vi "Open Me.vi"   [LabVIEW 2019]
uses:
  <userlib>/LevyLab/Instrument Framework/Instrument Types/Cryostat/Instrument.Cryostat.lvclass
  <userlib>/LevyLab/Lockin-Multichannel/Instrument.DAQ/Typedefs/Sweep.Configuration--Cluster.ctl
  <userlib>/LevyLab/Lockin-Multichannel/Instrument.DAQ/Typedefs/Sweep.Channel--Cluster--Array.ctl
  <userlib>/LevyLab/Lockin-Multichannel/Instrument.DAQ/Typedefs/Sweep.Channel--Cluster.ctl
  <userlib>/LevyLab/Lockin-Multichannel/Instrument.DAQ/Typedefs/Sweep.Pattern--Enum.ctl
  SweepControl/Typedefs/ScanControl.ctl
  SweepControl/Typedefs/Cluster - ScanControl.ctl
  SweepControl/Typedefs/Enum - Priority.ctl
  SweepControl/Typedefs/Enum - Action.ctl
  SweepControl/Typedefs/ScanParamters.ctl
  SweepControl/Typedefs/Cluster - ScanParamters.ctl
  SweepControl/Typedefs/PostAction.ctl
  SweepControl/Typedefs/Enum - PostAction.ctl
  Control Experiment/Control Experiment.lvclass/Control Experiment.ctl
  Transport/Transport.lvclass/Transport.ctl
  SweepControl/SweepControl.lvclass/SweepControl.ctl
  1ef964a1-2c2c-4dd9-a479-5e3cab6bfeb3.vi
  Control Experiment/subVIs/String Label.vi
  Transport/Transport.lvclass
  Control Experiment/Control Experiment.lvclass
  SweepControl/SweepControl.lvclass
  <userlib>/LevyLab/Lockin-Multichannel/Instrument.Lockin/Instrument.Lockin.lvclass
  <userlib>/LevyLab/Lockin-Multichannel/Instrument.DAQ/Instrument.DAQ.lvclass
panel:
  # "Open the block diagram"
types:
  T1 = typedef "SweepControl.lvclass/ScanParamters.ctl" = T2[]
  T2 = typedef "SweepControl.lvclass/Cluster - ScanParamters.ctl" = cluster{"Start":dbl, "End":dbl, "Step":dbl, "Rate":dbl, "Waveform type":enum16{"linear", "triangle", "power"}, "wait (ms or K)":dbl, "Address":string, "channel":i32}
  T3 = typedef "SweepControl.lvclass/ScanControl.ctl" = T4[]
  T4 = typedef "SweepControl.lvclass/Cluster - ScanControl.ctl" = cluster{"Priority":T5, "Scan name":T6}
  T5 = typedef "SweepControl.lvclass/Enum - Priority.ctl" = enum16{"Priority 0", "Priority 1", "Priority 2", "Priority 3", "Priority 4", "Priority 5"}
  T6 = typedef "SweepControl.lvclass/Enum - Action.ctl" = enum16{"OFF", "time", "Lockin Amplitude", "Lockin Frequency", "Lockin Bias", "Delay", "Strain", "DAQ Bias", "Magnet Field", "Temperature", "MW f1", "MW f2", "MW Amplitude1", "MW Amplitude2"}
  T7 = typedef "Instrument.DAQ.lvclass/Sweep.Configuration--Cluster.ctl" = cluster{"Sweep Time (s)":dbl, "Initial Wait (s)":dbl, "Return to Start":bool, "Channels":T8}
  T8 = typedef "Instrument.DAQ.lvclass/Sweep.Channel--Cluster--Array.ctl" = T9[]
  T9 = typedef "Instrument.DAQ.lvclass/Sweep.Channel--Cluster.ctl" = cluster{"Enable?":bool, "Channel":u16, "Start":dbl, "End":dbl, "Pattern":T10, "Table":dbl[]}
  T10 = typedef "Instrument.DAQ.lvclass/Sweep.Pattern--Enum.ctl" = enum16{"Ramp /", "Ramp /\\", "Smooth Ramp _/", "Smooth Ramp _/\\_", "Table"}
  T11 = typedef "SweepControl.lvclass/PostAction.ctl" = T12[]
  T12 = typedef "SweepControl.lvclass/Enum - PostAction.ctl" = enum16{"Do Nothing", "Wait (time)", "Wait (Temperature)", "Wait (<T ; B sweep)", "Wait (Magnet)"}
  T13 = typedef "Control Experiment.lvclass/Instrument Classes--cluster.ctl" = cluster{"KH7008":refnum<class "Instrument.KH7008.lvclass">[], "Lockin":refnum<class "Instrument.Lockin.lvclass">, "Temperature":refnum<class "Instrument.Cryostat.lvclass">, "Magnet":refnum<class "Instrument.Cryostat.lvclass">, "Rotator":refnum<class "Instrument.Cryostat.lvclass">, "Level":refnum<class "Instrument.Cryostat.lvclass">, "Capacitance Bridge":refnum<class "Instrument.CBridge.lvclass">, "Delay Line":refnum<class "Instrument.DelayLine.lvclass">, "Strain Cell":refnum<class "Instrument.Strain.lvclass">, "VNA":refnum<class "Instrument.VNA.lvclass">, "Voltage Source":refnum<class "Instrument.VSource.lvclass">}
  T14 = typedef "Instrument.DAQ.lvclass/PublicEvents--DAQ.getSweepWaveforms.ctl" = cluster{"AO_wfm":waveform(dbl)[], "AI_wfm":waveform(dbl)[], "X_wfm":waveform(dbl)[], "Y_wfm":waveform(dbl)[]}
  T15 = typedef "LV-Data.lvclass/Dictionary--cluster.ctl" = cluster{"key":string, "value":variant}
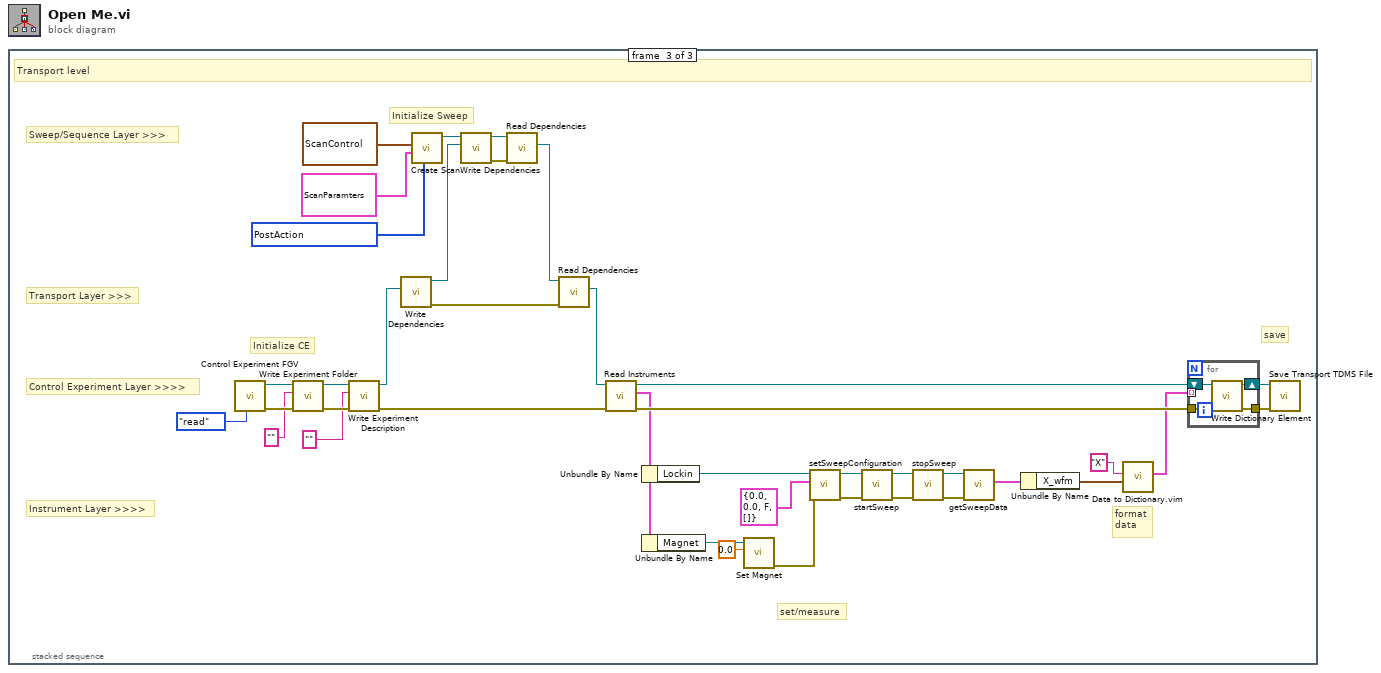
[diagram p0: block diagram]
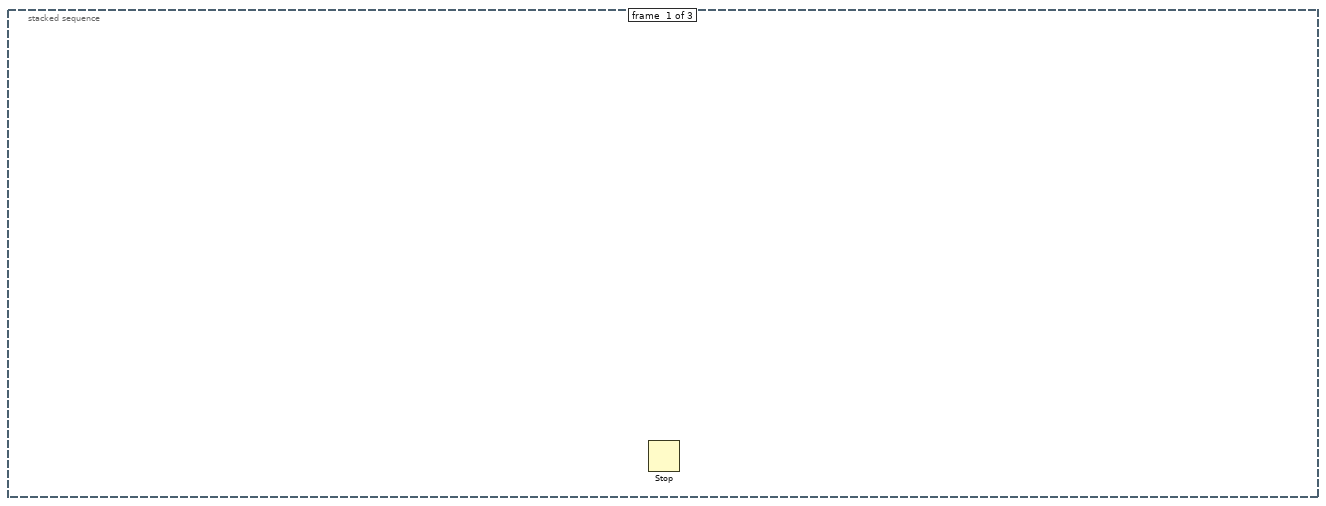
[diagram p2: hidden frame]
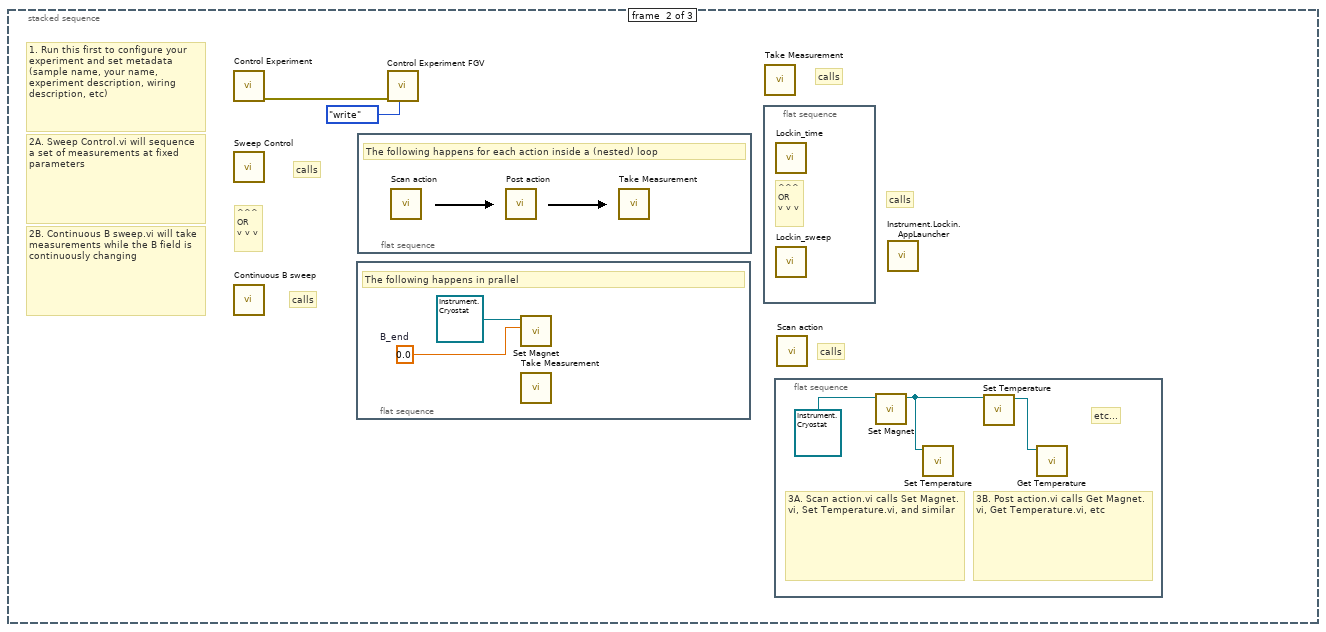
[diagram p3: hidden frame]
diagram:
  n1 = stacked-sequence {
    frame #0 {
      n2 = Stop() -> ()  [unwired: 1 in]
    }
    frame #1 {
      # "calls"
      # "calls"
      # "calls"
      # "calls"
      # "calls"
      # "^^^\nOR\nv v v"
      # "2A. Sweep Control.vi will sequence a set of measurements at fixed parameters"
      # "2B. Continuous B sweep.vi will take measurements while the B field is continuously changing"
      # "1. Run this first to configure your experiment and set metadata (sample name, your name, experiment description, wiring description, etc)"
      n3 = call "Control Experiment.vi"() -> ("Error Out"=w1:errorcluster)  [unwired: 11 in]
      n4 = call "Sweep Control.vi"() -> ()  [unwired: 11 in, 1 out]
      n5 = call "Continuous B sweep.vi"() -> ()  [unwired: 11 in, 1 out]
      n6 = flat-sequence {
        frame #0 {
          w6 = 0.0  # B_end
          # "The following happens in prallel"
          n7 = call-dynamic "Set Magnet.vi"("Target Field (T)"=w6, "Instrument.Cryostat in"=refnum<class "Instrument.Cryostat.lvclass"> refnum) -> ()  [unwired: 8 in, 2 out]
          n8 = call "Take Measurement.vi"() -> ()  [unwired: 10 in, 2 out]
        }
      }
      n9 = flat-sequence {
        frame #0 {
          # "The following happens for each action inside a (nested) loop"
          n10 = call "Scan action.vi"() -> ()  [unwired: 9 in, 3 out]
          n11 = call "Post action.vi"() -> ()  [unwired: 10 in, 2 out]
          n12 = call "Take Measurement.vi"() -> ()  [unwired: 10 in, 2 out]
        }
      }
      n13 = call "Control Experiment FGV.vi"("Function"=enum16{"read", "write"}."write", "error in (no error)"=w1) -> ()  [unwired: 8 in, 2 out]
      n14 = flat-sequence {
        frame #0 {
          # "^^^\nOR\nv v v"
          n15 = call "Lockin_time.vi"() -> ()  [unwired: 10 in, 2 out]
          n16 = call "Lockin_sweep.vi"() -> ()  [unwired: 9 in, 2 out]
        }
      }
      n17 = call "Take Measurement.vi"() -> ()  [unwired: 10 in, 2 out]
      n18 = flat-sequence {
        frame #0 {
          # "etc..."
          # "3B. Post action.vi calls Get Magnet.vi, Get Temperature.vi, etc"
          # "3A. Scan action.vi calls Set Magnet.vi, Set Temperature.vi, and similar"
          n19 = call-dynamic "Set Magnet.vi"("Instrument.Cryostat in"=refnum<class "Instrument.Cryostat.lvclass"> refnum) -> ("Instrument.Cryostat out"=w5:refnum<class "Instrument.Cryostat.lvclass">)  [unwired: 9 in, 1 out]
          n20 = call-dynamic "Set Temperature.vi"("Instrument.Cryostat in"=w5) -> ()  [unwired: 9 in, 2 out]
          n21 = call-dynamic "Set Temperature.vi"("Instrument.Cryostat in"=w5) -> ("Instrument.Cryostat out"=w4:refnum<class "Instrument.Cryostat.lvclass">)  [unwired: 9 in, 1 out]
          n22 = call-dynamic "Get Temperature.vi"("Instrument.Cryostat in"=w4) -> ()  [unwired: 6 in, 5 out]
        }
      }
      n23 = call "Scan action.vi"() -> ()  [unwired: 9 in, 3 out]
      n24 = call <userlib>:"Instrument.Lockin.AppLauncher.vi"() -> ()  [unwired: 12 in]
    }
    frame #2 {
      w14 = T11 [enum."Do Nothing", enum."Wait (Temperature)", enum."Do Nothing", enum."Do Nothing"] items=["Do Nothing", "Wait (time)", "Wait (Temperature)", "Wait (<T ; B sweep)", "Wait (Magnet)"] ("Post action (indexing priority)")
      # "save"
      # "format\ndata"
      # "set/measure"
      # "Initialize Sweep"
      # "Initialize CE"
      # "Instrument Layer >>>>"
      # "Control Experiment Layer >>>>"
      # "Transport Layer >>>"
      # "Sweep/Sequence Layer >>>"
      # "Transport level"
      n25 = call "Control Experiment FGV.vi"("Function"=enum16{"read", "write"}."read") -> ("error out"=w45:errorcluster, "Control Experiment.lvclass out"=w46:refnum<class "Control Experiment.lvclass">)  [unwired: 9 in]
      n26 = call "Write Experiment Folder.vi"("error in (no error)"=w45, "Experiment Folder"="", "Control Experiment in"=w46) -> ("error out"=w43:errorcluster, "Control Experiment out"=w44:refnum<class "Control Experiment.lvclass">)  [unwired: 7 in]
      n27 = call "Write Experiment Description.vi"("error in (no error)"=w43, "Experiment Description"="", "Control Experiment in"=w44) -> ("error out"=w24:errorcluster, "Control Experiment out"=w31:refnum<class "Control Experiment.lvclass">)  [unwired: 7 in]
      n28 = call "Write Dependencies.vi"("Control Experiment"=w31) -> ("error out"=w22:errorcluster, "Transport out"=w30:refnum<class "Transport.lvclass">)  [unwired: 9 in]
      n29 = call "Create Scan.vi"("Post action (indexing priority)"=w14, "Scan parameters"=T1 [{"Start"=0.14, "End"=-0.060000000000000005, "Step"=-0.060000000000000005, "Rate"=0.0, "Waveform type"=enum."linear", "wait (ms or K)"=10000.0, "Address"="Dev2/ao0", "channel"=1}, {"Start"=0.14, "End"=-0.060000000000000005, "Step"=-0.060000000000000005, "Rate"=0.0, "Waveform type"=enum."linear", "wait (ms or K)"=10000.0, "Address"="Dev2/ao0", "channel"=1}, {"Start"=0.14, "End"=-0.060000000000000005, "Step"=-0.060000000000000005, "Rate"=0.0, "Waveform type"=enum."linear", "wait (ms or K)"=10000.0, "Address"="Dev2/ao0", "channel"=1}, {"Start"=0.14, "End"=-0.060000000000000005, "Step"=-0.060000000000000005, "Rate"=0.0, "Waveform type"=enum."linear", "wait (ms or K)"=10000.0, "Address"="Dev2/ao0", "channel"=1}], "Scan control"=T3 [{"Priority"=enum."Priority 1", "Scan name"=enum."Lockin Amplitude"}, {"Priority"=enum."Priority 2", "Scan name"=enum."Lockin Bias"}, {"Priority"=enum."Priority 0", "Scan name"=enum."Delay"}, {"Priority"=enum."Priority 2", "Scan name"=enum."Magnet Field"}]) -> ("SweepControl"=w17:refnum<class "SweepControl.lvclass">)  [unwired: 8 in]
      n30 = call "Write Dependencies.vi"("Transport"=w30, "SweepControl in"=w17) -> ("error out"=w21:errorcluster, "SweepControl out"=w29:refnum<class "SweepControl.lvclass">)  [unwired: 8 in]
      n31 = call "Read Dependencies.vi"("error in (no error)"=w21, "SweepControl in"=w29) -> ("Transport"=w28:refnum<class "Transport.lvclass">)  [unwired: 7 in, 2 out]
      n32 = call "Read Dependencies.vi"("error in (no error)"=w22, "Transport"=w28) -> ("C.E."=w39:refnum<class "Control Experiment.lvclass">)  [unwired: 7 in, 2 out]
      n33 = call "Read Instruments.vi"("error in (no error)"=w24, "Control Experiment in"=w39) -> ("error out"=w23:errorcluster, "Instruments"=w20:T13, "Control Experiment out"=w25:refnum<class "Control Experiment.lvclass">)  [unwired: 7 in]
      n34 = Unbundle By Name(w20) -> ("Lockin"=w38:refnum<class "Instrument.Lockin.lvclass">)
      n35 = Unbundle By Name(w20) -> ("Magnet"=w19:refnum<class "Instrument.Cryostat.lvclass">)
      n36 = call-dynamic "Set Magnet.vi"("Target Field (T)"=0.0, "Instrument.Cryostat in"=w19) -> ("error out"=w12:errorcluster)  [unwired: 8 in, 1 out]
      n37 = call <userlib>:"setSweepConfiguration.vi"("error in (no error)"=w12, "Configure Sweep"=T7 {"Sweep Time (s)"=0.0, "Initial Wait (s)"=0.0, "Return to Start"=FALSE, "Channels"=[]}, "Instrument.Lockin in"=w38) -> ("error out"=w37:errorcluster, "Instrument.Lockin out"=w36:refnum<class "Instrument.Lockin.lvclass">)  [unwired: 7 in]
      n38 = call <userlib>:"startSweep.vi"("error in (no error)"=w37, "Instrument.Lockin in"=w36) -> ("error out"=w35:errorcluster, "Instrument.Lockin out"=w34:refnum<class "Instrument.Lockin.lvclass">)  [unwired: 8 in]
      n39 = call <userlib>:"stopSweep.vi"("error in (no error)"=w35, "Instrument.Lockin in"=w34) -> ("error out"=w33:errorcluster, "Instrument.Lockin out"=w32:refnum<class "Instrument.Lockin.lvclass">)  [unwired: 8 in]
      n40 = call <userlib>:"getSweepData.vi"("error in (no error)"=w33, "Instrument.Lockin in"=w32) -> ("Data out"=w13:T14)  [unwired: 7 in, 2 out]
      n41 = Unbundle By Name(w13) -> ("X_wfm"=w11:waveform(dbl)[])
      n42 = call "Data to Dictionary.vim"("Data in"=w11, "Label in"="X" ("Input String")) -> ("Data out"=w9:T15[])  [unwired: 8 in, 1 out]
      n43 = for {
        tunnel: w9 -> [_] mode=indexing
        shift-right: [w50] -> w27
        shift-left: w25 -> [w48]
        tunnel: w23 -> [w47]
        tunnel: [w49] -> w26
        n44 = call "Write Dictionary Element.vi"("error in (no error)"=w47, "Control Experiment in"=w48) -> ("error out"=w49:errorcluster, "Control Experiment out"=w50:refnum<class "Control Experiment.lvclass">)  [unwired: 8 in]
      }
      n45 = call "Save Transport TDMS File.vi"("error in (no error)"=w26, "Control Experiment in"=w27) -> ()  [unwired: 8 in, 2 out]
    }
  }
